vi "writeToXML.vi"(8 "error in (no error)":errorcluster, 10 "ClassLabel":string, 11 "TCSWFSStatus in":refnum<class "TCSWFSStatus.lvclass">) -> (0 "error out":errorcluster, 2 "XMLout":string, 3 "TCSWFSStatus out":refnum<class "TCSWFSStatus.lvclass">)   [LabVIEW 2014, in "TCSDataDefinitions.lvlib" / "TCSWFSStatus.lvlib" / "TCSWFSStatus.lvclass"]
uses:
  TCSWFSStatus.lvclass
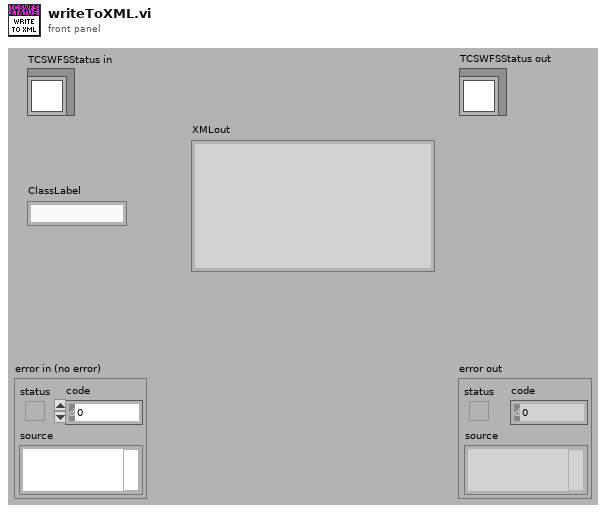
[diagram p1: front panel]
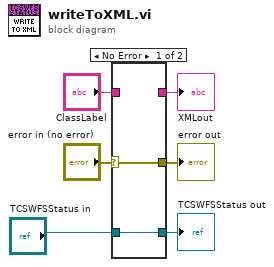
[diagram p0: block diagram]
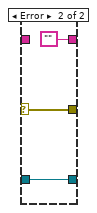
[diagram p2: hidden frame]
diagram:
  n1 = case shown="No Error" "error in (no error)" {
    selector: "error in (no error)" -> [w7 w11]
    tunnel: [w7 w11] -> w5
    tunnel: [w8 w10] -> w4
    tunnel: "TCSWFSStatus in" -> [w8 w10]
    tunnel: [_ ""] -> w3
    tunnel: "ClassLabel" -> [_ _]
    frame No Error {
    }
    frame Error {
    }
  }
  "error out" <- w5
  "TCSWFSStatus out" <- w4
  "XMLout" <- w3
